vi "test Disabled Device Can Be Deployed.vi"(8 "error in (no error)":errorcluster, 11 "TestCase in":refnum<class "Disabled Custom Device.lvclass">) -> (0 "error out":errorcluster, 3 "TestCase out":refnum<class "Disabled Custom Device.lvclass">)   [LabVIEW 2024, in "Disabled Custom Device.lvclass"]
uses:
  Disabled Custom Device.lvclass
  Disabled Custom Device.lvclass/Disabled Custom Device.ctl
  <vilib>/addons/_JKI Toolkits/VI Tester/TestCase.llb/TestCase.lvclass
  C:/Program Files/National Instruments/LabVIEW 2024/vi.lib/addons/_JKI Toolkits/VI Tester/TestCase.llb/TestCase.lvclass
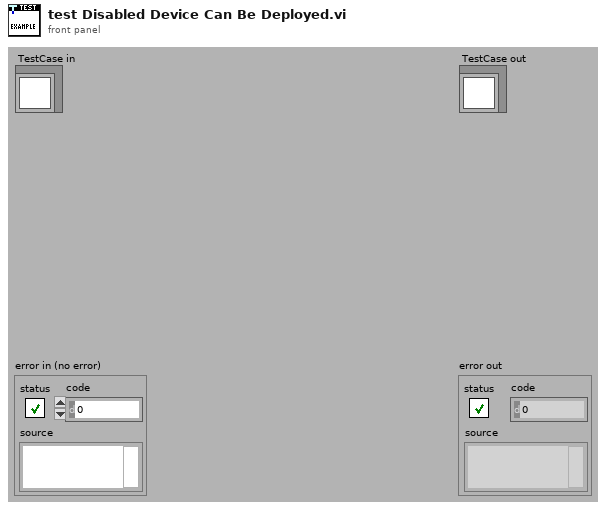
[diagram p1: front panel]
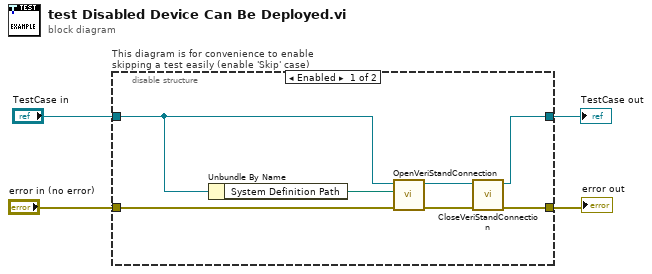
[diagram p0: block diagram]
diagram:
  n1 = disable-structure "This diagram is for convenience to enable skipping a test easily (enable 'Skip' case)" shown="Enabled" {
    disable-tunnel: "TestCase in" -> [w6 w15]
    disable-tunnel: [w7 w13] -> w1
    disable-tunnel: [w8 w14] -> w3
    disable-tunnel: "error in (no error)" -> [w11 w12]
    frame Enabled {
      n2 = Unbundle By Name(w6) -> ("System Definition Path"=w5:path)
      n3 = call-dynamic "OpenVeriStandConnection.vi"("error in (no error)"=w11, "System Definition File"=w5, "VeriStand Test Case in"=w6) -> ("error out"=w10:errorcluster, "VeriStand Test Case out"=w9:refnum<class "Disabled Custom Device.lvclass">)  [unwired: 6 in, 1 out]
      n4 = call-dynamic "CloseVeriStandConnection.vi"("error in (no error)"=w10, "VeriStand Test Case in"=w9) -> ("error out"=w8:errorcluster, "VeriStand Test Case out"=w7:refnum<class "Disabled Custom Device.lvclass">)  [unwired: 8 in]
    }
    frame Disabled {
      # "skip test result while test is under development"
      n5 = call <vilib>:"skip.vi"("error in (no error)"=w12, "TestCase in"=w15) -> ("error out"=w14:errorcluster, "TestCase out"=w13:refnum<class "Disabled Custom Device.lvclass">)  [unwired: 8 in]
    }
  }
  "error out" <- w3
  "TestCase out" <- w1
